vi "save channels to interleaved multi-tiff files.vi"(8 "frame number in":i32, 9 "last frame":bool, 11 "image data in":dbl[][](array[numeric])) -> ()   [LabVIEW 2012]
doc: "SciScan 1.2 160622"
uses:
  Custom Controls/file format type def.ctl
  GFG/GFGpathGet.vi
  GFG/GFGnumericGet.vi
  GFG/GFGstringGet.vi
  Libtiff3/libtiff3.llb/libtiff3.lvlib
  GFG/GFG library.lvlib
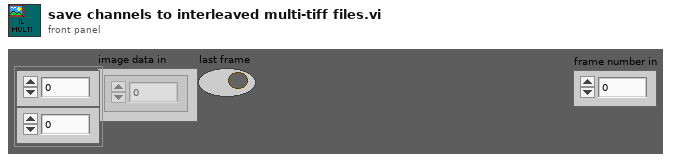
[diagram p1: front panel]
types:
  T1 = typedef "file format type def.ctl" = enum16{"16bit raw", "32bit raw", "16bit multi-tiff (interleave)", "16bit multi-tiff (separate)", "16bit multi-tiff (stacked)", "32bit multi-tiff (interleave)", "32bit multi-tiff (separate)", "32bit multi-tiff (stacked)", "16bit tiff series (interleave)", "16bit tiff series (separate)", "16bit tiff series (stacked)", "32bit tiff series (interleave)", "32bit tiff series (separate)", "32bit tiff series (stacked)"}
  T2 = cluster{"no..of.frames.to.acquire":dbl, "x.pixels":dbl, "y.pixels":dbl, "x.pixel.sz":dbl, "y.pixel.sz":dbl}
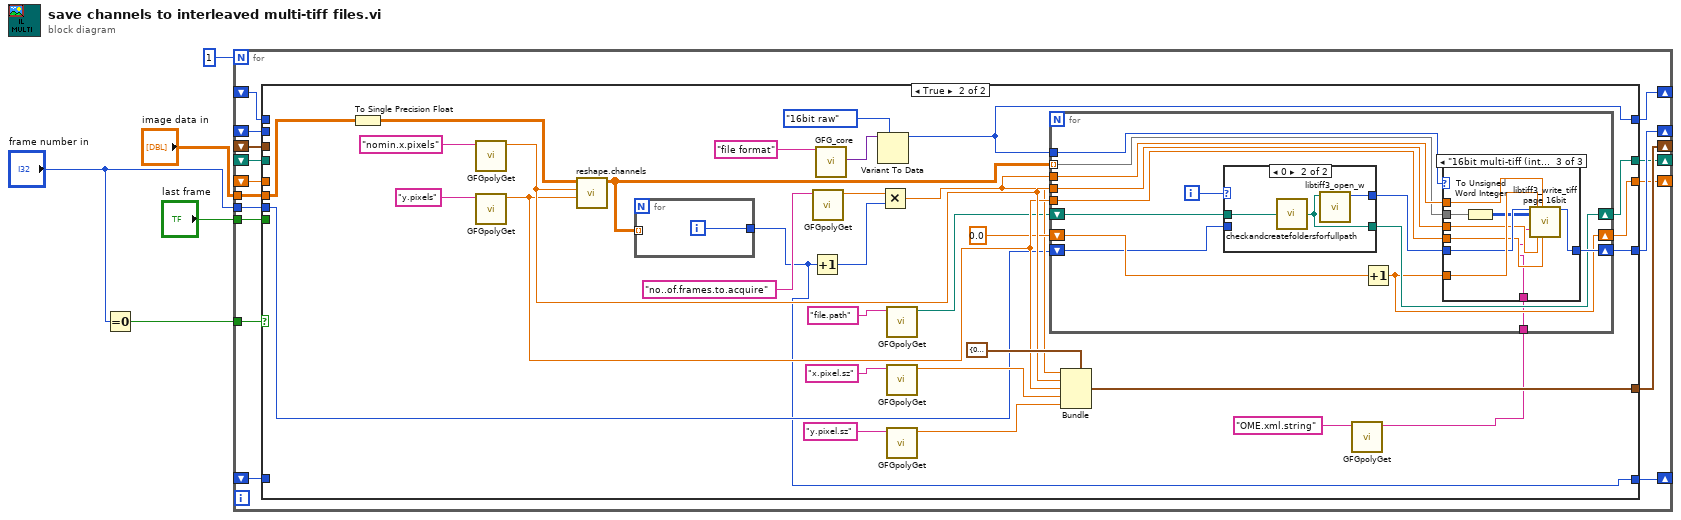
[diagram p0: block diagram]
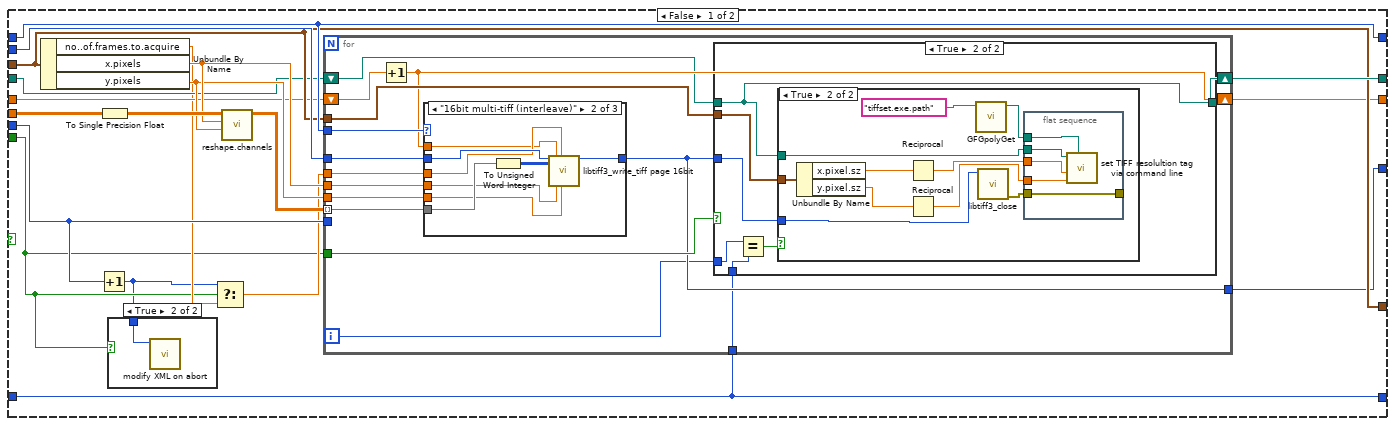
[diagram p2: hidden frame]
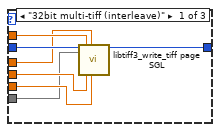
[diagram p4: hidden frame]
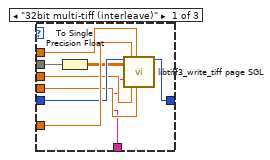
[diagram p9: hidden frame]
diagram:
  n1 = Equal To 0?(x="frame number in") -> (x = 0?=w4:bool)
  n2 = for {
    N: 1 -> [_]
    tunnel: w4 -> [w21]
    shift-right: [w20] -> _
    shift-left: _ -> [w19]
    tunnel: "image data in" -> [w18]
    shift-right: [w17] -> _
    shift-left: _ -> [w16]
    shift-right: [w15] -> _
    shift-left: _ -> [w14]
    shift-right: [w13] -> _
    shift-left: _ -> [w12]
    tunnel: "last frame" -> [w11]
    tunnel: "frame number in" -> [w10]
    shift-right: [w9] -> _
    shift-left: _ -> [w8]
    shift-right: [w7] -> _
    shift-left: _ -> [w6]
    n3 = case shown="True" w21 {
      tunnel: w16 -> [w38 _]
      tunnel: [w36 w110] -> w20
      tunnel: w19 -> [w40 _]
      tunnel: w18 -> [w35 w106]
      tunnel: [w38 w112] -> w17
      tunnel: [w37 w113] -> w15
      tunnel: w14 -> [w37 _]
      tunnel: [w39 w105] -> w13
      tunnel: w12 -> [w28 _]
      tunnel: w11 -> [w23 _]
      tunnel: w10 -> [w26 w100]
      tunnel: [w29 w103] -> w9
      tunnel: w8 -> [w30 _]
      tunnel: [w27 w97] -> w7
      tunnel: w6 -> [w27 _]
      frame False {
        n4 = Unbundle By Name(w37) -> ("no..of.frames.to.acquire"=w25:dbl, "x.pixels"=w32:dbl, "y.pixels"=w31:dbl)
        n5 = Increment(x=w26) -> (x+1=w22:i32)
        n6 = To Single Precision Float(number=w35) -> (single precision float=w34:sgl[][])
        n7 = case shown="True" w23 {
          tunnel: w22 -> [_ w41]
          frame False {
          }
          frame True {
            n8 = call "modify XML on abort.vi"("frame number"=w41) -> ()  [unwired: 10 in, 1 out]
          }
        }
        n9 = Select(t=w22, s=w23, f=w25) -> (s? t:f=w24:dbl)
        n10 = call "reshape.channels.vi"("y.pixels"=w31, "x.pixels"=w32, "element"=w34) -> ("Array"=w33:dbl[][][])  [unwired: 8 in]
        n11 = for {
          tunnel: w23 -> [w56]
          tunnel: w33 -> [w55] mode=indexing
          tunnel: w40 -> [w54]
          tunnel: w24 -> [w52]
          tunnel: w26 -> [_]
          tunnel: w32 -> [w51]
          tunnel: w31 -> [w50]
          tunnel: w38 -> [w49]
          tunnel: w37 -> [w48]
          tunnel: [w47] -> w36
          shift-right: [w45] -> w29
          shift-left: w30 -> [w46]
          shift-right: [w53] -> w39
          shift-left: w28 -> [w44]
          tunnel: w27 -> [w43]
          i -> [w42]
          n12 = Increment(x=w46) -> (x+1=w45:dbl)
          n13 = case shown="\"16bit multi-tiff (interleave)\"" w49 {
            tunnel: w55 -> [w57 w71 _]
            tunnel: w54 -> [w63 w69 w72]
            tunnel: [w60 w68 w72] -> w47
            tunnel: w52 -> [w61 w67 _]
            tunnel: w45 -> [w62 w66 _]
            tunnel: w51 -> [w59 w65 _]
            tunnel: w50 -> [w58 w64 _]
            frame "32bit multi-tiff (interleave)" {
              n14 = call "libtiff3_write_tiff page SGL.vi"("Handle"=w63, "Image Pixels (Float)"=w57, "page"=w62, "x.pixels"=w59, "totalpages"=w61, "y.pixels"=w58) -> ("Handle out"=w60:i32)  [unwired: 12 in, 1 out]
            }
            frame "16bit multi-tiff (interleave)" {
              n15 = To Unsigned Word Integer(number=w71) -> (unsigned 16bit integer=w70:u16[][])
              n16 = call "libtiff3_write_tiff page 16bit.vi"("Handle"=w69, "Image Pixels (U16)"=w70, "page"=w66, "x.pixels"=w65, "totalpages"=w67, "y.pixels"=w64) -> ("Handle out"=w68:i32)  [unwired: 12 in, 1 out]
            }
            frame Default {
            }
          }
          n17 = case shown="True" w56 {
            tunnel: w48 -> [_ w79]
            tunnel: w44 -> [w73 w74]
            tunnel: w47 -> [_ w78]
            tunnel: [w73 w74] -> w53
            tunnel: w43 -> [_ w75]
            tunnel: w42 -> [_ w76]
            frame False {
            }
            frame True {
              n18 = Equal?(x=w76, y=w75) -> (x = y?=w77:bool)
              n19 = case shown="True" w77 {
                tunnel: w79 -> [_ w84]
                tunnel: w74 -> [_ w83]
                tunnel: w78 -> [_ w80]
                frame False {
                }
                frame True {
                  n20 = Unbundle By Name(w84) -> ("x.pixel.sz"=w85:dbl, "y.pixel.sz"=w86:dbl)
                  n21 = Reciprocal(x=w85) -> (1/x=w87:dbl)
                  n22 = Reciprocal(x=w86) -> (1/x=w88:dbl)
                  n23 = call-poly "GFGpolyGet.vi"("Variable Name in"="tiffset.exe.path") -> ("Path"=w81:path)  [unwired: 8 in, 2 out]
                  n24 = call "libtiff3_close.vi"("Handle"=w80) -> ("error out"=w89:errorcluster)  [unwired: 9 in]
                  n25 = flat-sequence {
                    tunnel: w83 -> [w90]
                    tunnel: w89 -> [w92]
                    tunnel: w87 -> [w94]
                    tunnel: w88 -> [w93]
                    tunnel: w81 -> [w91]
                    tunnel: [w92] -> _
                    frame #0 {
                      n26 = call "set TIFF resolultion tag via command line.vi"("tiffset.exe file path"=w91, "y pixels per m"=w93, "x pixels per m"=w94, "TIFF file path"=w90) -> ()  [unwired: 8 in]
                    }
                  }
                }
              }
            }
          }
        }
      }
      frame True {
        n27 = To Single Precision Float(number=w106) -> (single precision float=w109:sgl[][])
        n28 = call-poly "GFGpolyGet.vi"("Variable Name in"="nomin.x.pixels" ("Tag in")) -> ("Numeric"=w108:dbl)  [unwired: 8 in, 2 out]
        n29 = call-poly "GFGpolyGet.vi"("Variable Name in"="y.pixels" ("Tag in")) -> ("Numeric"=w107:dbl)  [unwired: 8 in, 2 out]
        n30 = call "reshape.channels.vi"("y.pixels"=w107, "x.pixels"=w108, "element"=w109) -> ("Array"=w102:dbl[][][])  [unwired: 8 in]
        n31 = for {
          tunnel: w102 -> [_] mode=indexing
          tunnel: [w126] -> w97
          i -> [w126]
        }
        n32 = Increment(x=w97) -> (x+1=w98:i32)
        n33 = call-poly "GFGpolyGet.vi"("Variable Name in"="no..of.frames.to.acquire") -> ("Numeric"=w111:dbl)  [unwired: 8 in, 2 out]
        n34 = call "GFG_core.vi"("Variable Name in"="file format") -> ("Variant Out"=w124:variant)  [unwired: 12 in, 6 out]
        n35 = Variant To Data(type=file_format_type_def."16bit raw" ("file format"), Variant=w124) -> (data=w112:T1)  [unwired: 1 in, 1 out]
        n36 = Multiply(x=w111, y=w98) -> (x*y=w101:dbl)
        n37 = call-poly "GFGpolyGet.vi"("Variable Name in"="file.path") -> ("Path"=w99:path)  [unwired: 8 in, 2 out]
        n38 = call-poly "GFGpolyGet.vi"("Variable Name in"="x.pixel.sz" ("Tag in")) -> ("Numeric"=w116:dbl)  [unwired: 8 in, 2 out]
        n39 = call-poly "GFGpolyGet.vi"("Variable Name in"="y.pixel.sz" ("Tag in")) -> ("Numeric"=w115:dbl)  [unwired: 8 in, 2 out]
        n40 = Bundle(cluster=T2 {"no..of.frames.to.acquire"=0.0, "x.pixels"=0.0, "y.pixels"=0.0, "x.pixel.sz"=0.0, "y.pixel.sz"=0.0} ("output cluster"), "no..of.frames.to.acquire"=w101, "x.pixels"=w108, "y.pixels"=w107, "x.pixel.sz"=w116, "y.pixel.sz"=w115) -> (w113:T2)
        n41 = call-poly "GFGpolyGet.vi"("Variable Name in"="OME.xml.string" ("Tag in")) -> ("String"=w95:string)  [unwired: 9 in, 1 out]
        n42 = for {
          tunnel: w112 -> [w140]
          tunnel: w101 -> [w139]
          tunnel: w108 -> [w137]
          tunnel: w107 -> [w136]
          tunnel: w102 -> [w135] mode=indexing
          shift-right: [w131] -> w103
          shift-left: 0.0 -> [w132]
          shift-right: [w138] -> w110
          shift-left: w100 -> [w129]
          shift-right: [w133] -> w105
          shift-left: w99 -> [w128]
          tunnel: w95 -> [w127]
          i -> [w130]
          n43 = case shown="0" w130 {
            tunnel: [w141 w145] -> w134
            tunnel: [w142 w144] -> w133
            tunnel: w128 -> [w142 w143]
            tunnel: w129 -> [w141 _]
            frame 1, Default {
            }
            frame 0 {
              n44 = call "checkandcreatefoldersforfullpath.vi"("Path IN"=w143) -> ("Path OUT"=w144:path)  [unwired: 4 in]
              n45 = call "libtiff3_open_w.vi"("Input path"=w144) -> ("handle"=w145:i32)  [unwired: 9 in, 1 out]
            }
          }
          n46 = Increment(x=w132) -> (x+1=w131:dbl)
          n47 = case shown="\"16bit multi-tiff (interleave)\"" w140 {
            tunnel: w135 -> [w150 _ w161]
            tunnel: w134 -> [w151 w155 w162]
            tunnel: w131 -> [w152 _ w163]
            tunnel: w139 -> [w153 _ w164]
            tunnel: [w154 w155 w157] -> w138
            tunnel: w137 -> [w147 _ w159]
            tunnel: w136 -> [w148 _ w158]
            tunnel: w127 -> [w146 _ w156]
            frame "32bit multi-tiff (interleave)" {
              n48 = To Single Precision Float(number=w150) -> (single precision float=w149:sgl[][])
              n49 = call "libtiff3_write_tiff page SGL.vi"("Handle"=w151, "Image Pixels (Float)"=w149, "Image Description"=w146, "page"=w152, "x.pixels"=w147, "totalpages"=w153, "y.pixels"=w148) -> ("Handle out"=w154:i32)  [unwired: 11 in, 1 out]
            }
            frame Default {
            }
            frame "16bit multi-tiff (interleave)" {
              n50 = To Unsigned Word Integer(number=w161) -> (unsigned 16bit integer=w160:u16[][])
              n51 = call "libtiff3_write_tiff page 16bit.vi"("Handle"=w162, "Image Pixels (U16)"=w160, "ImageDescription"=w156, "page"=w163, "x.pixels"=w159, "totalpages"=w164, "y.pixels"=w158) -> ("Handle out"=w157:i32)  [unwired: 11 in, 1 out]
            }
          }
        }
      }
    }
  }
